vi "read_multipart.vi"(0 "zmq_mlt in":refnum<class "zmq_multipart_lib.lvclass">, 9 "timeout (ms)":u32=100, 11 "error in (no error)":errorcluster) -> (4 "zmq_mlt out":refnum<class "zmq_multipart_lib.lvclass">, 6 "multipart message DVR":refnum<data-value>, 8 "valid message":bool, 10 "timeout?":bool, 15 "error out":errorcluster)   [LabVIEW 2019, in "zmq_multipart_lib.lvlib" / "zmq_multipart_lib.lvclass"]
uses:
  zmq_multipart_lib.lvclass
  zmq_multipart_lib.lvclass/zmq_multipart_lib.ctl
  <vilib>/addons/zeromq/zmq_socket.lvclass
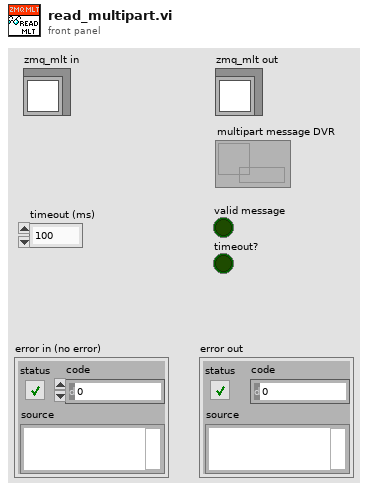
[diagram p1: front panel]
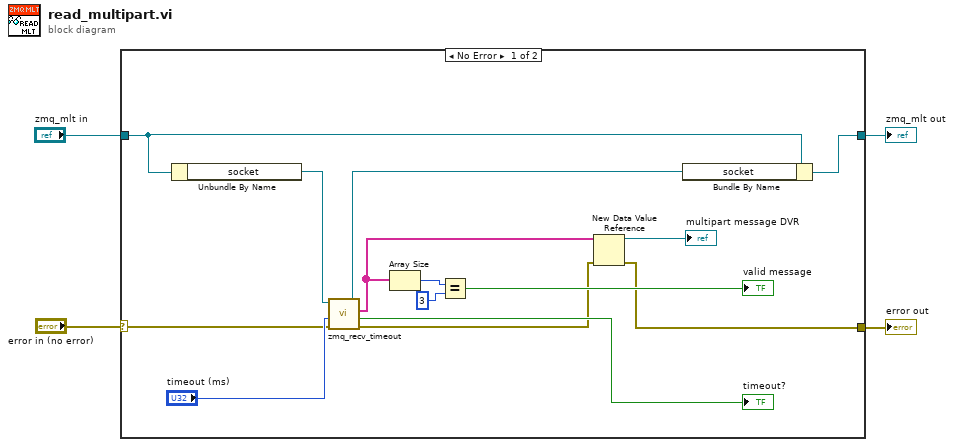
[diagram p0: block diagram]
diagram:
  n1 = case shown="No Error" "error in (no error)" {
    selector: "error in (no error)" -> [w14 w20]
    tunnel: [w5 w20] -> w4
    tunnel: "zmq_mlt in" -> [w18 w19]
    tunnel: [w17 w19] -> w2
    frame No Error {
      n2 = Unbundle By Name(w18) -> ("socket"=w13:refnum<class "zmq_socket.lvclass">)
      n3 = call <vilib>:"zmq_recv_timeout.vi"("error in"=w14, "timeout (ms)"="timeout (ms)", "socket in"=w13) -> ("error out"=w6:errorcluster, "timeout?"=→"timeout?":bool, "parts"=w8:string[], "socket out"=w9:refnum<class "zmq_socket.lvclass">)  [unwired: 1 in]
      n4 = Array Size(array=w8) -> (size(s)=w12:i32)
      n5 = Equal?(x=w12, y=3) -> (x = y?=→"valid message":bool)
      n6 = New Data Value Reference(data value=w8, error in=w6) -> (data value reference=→"multipart message DVR":refnum<data-value>, error out=w5:errorcluster)
      n7 = Bundle By Name(cluster=w18, "socket"=w9) -> (w17:refnum<class "zmq_multipart_lib.lvclass">)
    }
    frame Error {
    }
  }
  "error out" <- w4
  "zmq_mlt out" <- w2
